vi "Entry.vi"(8 "error in (no error)":errorcluster, 11 "New State":refnum<class "State Machine.lvclass">) -> (0 "error out":errorcluster, 3 "State out":refnum<class "State Machine.lvclass">)   [LabVIEW 2013, in "State Machine.lvclass"]
doc: "This is an abstract method. Override this method to define the behavior when you enter the state."
uses:
  State Machine.lvclass
  <vilib>/ni/Actors/State Actor/State Actor/State Actor.lvclass
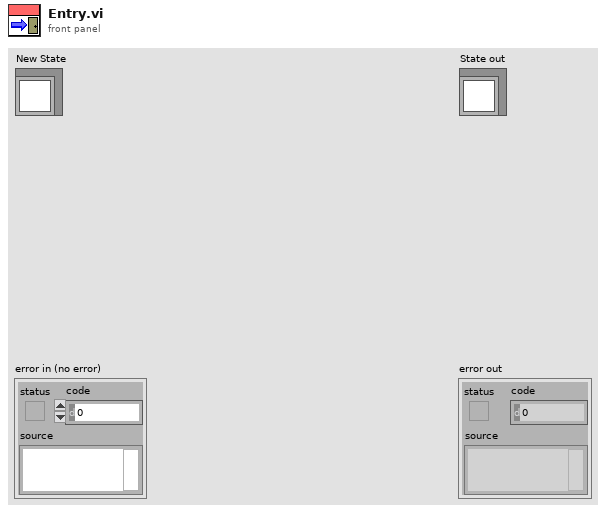
[diagram p1: front panel]
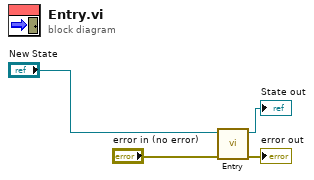
[diagram p0: block diagram]
diagram:
  n1 = call-parent "Entry.vi"("error in (no error)"="error in (no error)", "New State"="New State") -> ("error out"=→"error out":errorcluster, "State out"=→"State out":refnum<class "State Machine.lvclass">)  [unwired: 8 in]
